vi "Save New VI From XML.vi"(7 "Use VTT?":bool, 8 "error in (no error)":errorcluster, 9 "Block Diagram XML/VTT":string, 10 "Front Panel XML/VTT":string, 11 "Resources":T1[](array[typedef])) -> (0 "error out":errorcluster, 3 "Unique Temporary File Path":path)   [LabVIEW 2026, in "VILab.lvlib"]
uses:
  VILab.lvlib
  CTLs/Resource.ctl
  Find Resource by Type (String).vi
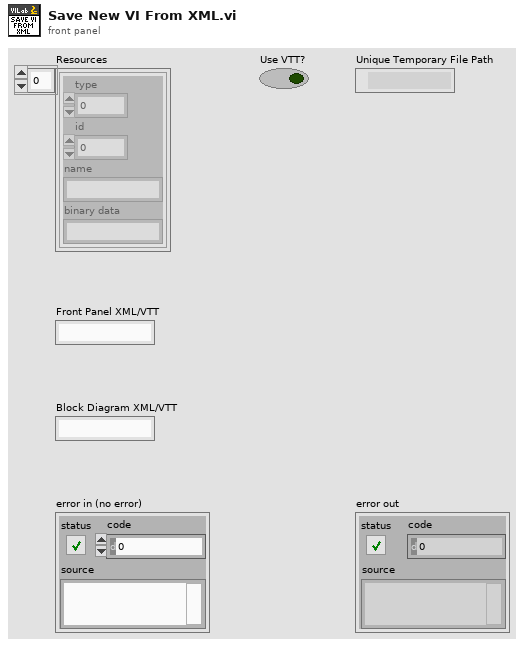
[diagram p1: front panel]
types:
  T1 = typedef "VILab.lvlib/Resource.ctl" = cluster{"type":u32, "id":i32, "name":string, "binary data":string}
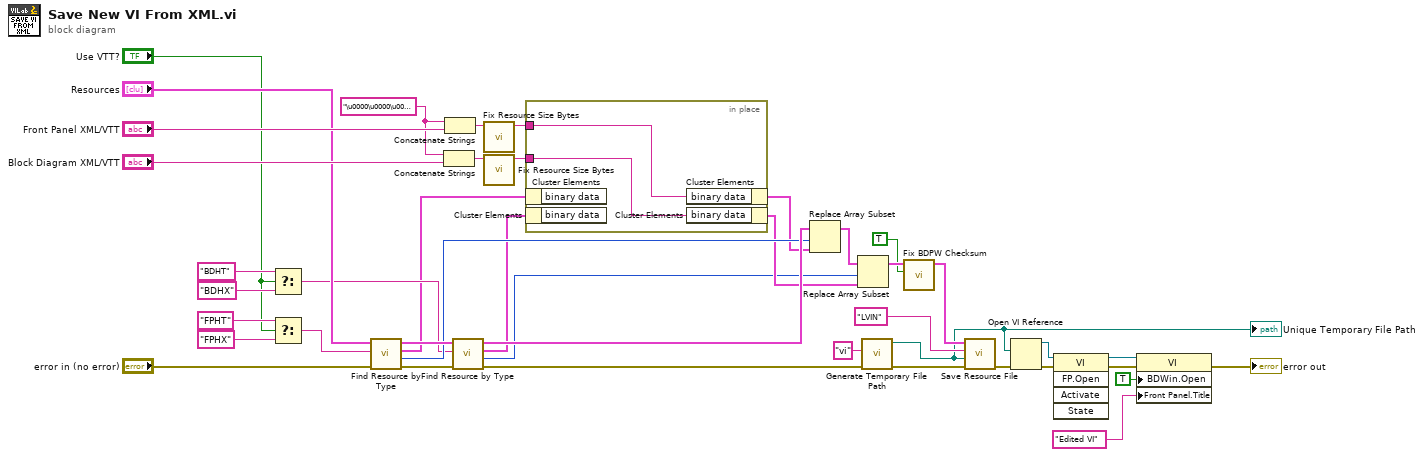
[diagram p0: block diagram]
diagram:
  w38 = "\u0000\u0000\u0000\u0000"
  n1 = Select(t="BDHT", s="Use VTT?", f="BDHX") -> (s? t:f=w4:string)
  n2 = Select(t="FPHT", s="Use VTT?", f="FPHX") -> (s? t:f=w12:string)
  n3 = call-poly "Find Resource by Type.vi"("error in (no error)"="error in (no error)", "Resource Type"=w12, "Resources"="Resources") -> ("error out"=w7:errorcluster, "Index"=w33:i32, "Resource"=w1:T1, "Resources out"=w41:T1[])  [unwired: 4 in, 1 out]
  n4 = Concatenate Strings(w38, "Block Diagram XML/VTT") -> (w36:string)
  n5 = Concatenate Strings(w38, "Front Panel XML/VTT") -> (w37:string)
  n6 = call-poly "Find Resource by Type.vi"("error in (no error)"=w7, "Resource Type"=w4, "Resources"=w41) -> ("error out"=w8:errorcluster, "Index"=w30:i32, "Resource"=w2:T1, "Resources out"=w42:T1[])  [unwired: 4 in, 1 out]
  n7 = call "Fix Resource Size Bytes.vi"("Data in"=w37) -> ("Data out"=w35:string)  [unwired: 10 in]
  n8 = call "Fix Resource Size Bytes.vi"("Data in"=w36) -> ("Data out"=w34:string)  [unwired: 10 in]
  n9 = in-place {
    in-place-border: w35 -> [w44]
    in-place-border: w34 -> [w43]
    n10 = in-place-cluster #1(w1) -> ()  [unwired: 1 out]
    n11 = in-place-cluster #2(w2) -> ()  [unwired: 1 out]
    n12 = in-place-cluster #1("binary data"=w44) -> (w32:T1)
    n13 = in-place-cluster #2("binary data"=w43) -> (w31:T1)
  }
  n14 = Replace Array Subset(array=w42, new element=w32, index=w33) -> (w29:T1[])
  n15 = Replace Array Subset(array=w29, new element=w31, index=w30) -> (w22:T1[])
  n16 = call <vilib>:"Generate Temporary File Path.vi"("error in (no error)"=w8, "Temporary File Extension (tmp)"="vi") -> ("error out"=w10:errorcluster, "Unique Temporary File Path"=w9:path)  [unwired: 8 in]
  "Unique Temporary File Path" <- w9
  n17 = call "Fix BDPW Checksum.vi"("Only fix 3rd hash (F)"=TRUE, "Resources"=w22) -> ("Resources out"=w21:T1[])  [unwired: 8 in, 1 out]
  n18 = call "Save Resource File.vi"("error in (no error)"=w10, "Path"=w9, "File type"="LVIN", "Resources"=w21) -> ("error out"=w27:errorcluster)  [unwired: 7 in]
  n19 = Open VI Reference(vi path=w9, error in (no error)=w27) -> (vi reference=w23:refnum<vi>, error out=w19:errorcluster)  [unwired: 4 in]
  n20 = invoke class="VI" method="FP.Open"(reference=w23, error in=w19) -> (reference out=w24:refnum<vi>, error out=w18:errorcluster)  [unwired: 3 in, 3 out]
  n21 = property class="VI"(reference=w24, error in=w18, "BDWin.Open"=TRUE ("Block Diagram Window:Open"), "Front Panel.Title"="Edited VI") -> (error out=→"error out":errorcluster)  [unwired: 1 out]
